vi "Add Round Key.vi"(0 "ExpandedKey(w)":u32[][](array[numeric]), 2 "Nb":i32=4, 7 "State.In":u16[][](array[numeric]), 9 "rnd (0)":i32, 11 "error in":errorcluster) -> (8 "State.Out":u16[][](array[numeric]), 15 "error out":errorcluster)   [LabVIEW 2020, in "Advanced Encryption Standard (AES).lvlib"]
doc: "In the AddRoundKey step, the subkey is combined with the state. For each round, a subkey is derived from the main key using Rijndael's key schedule; each subkey is the same size as the state. The subkey is added by combining each byte of the state with the corresponding byte of the subkey using bitwise XOR.\n\n<inline>"
uses:
  Advanced Encryption Standard (AES).lvlib
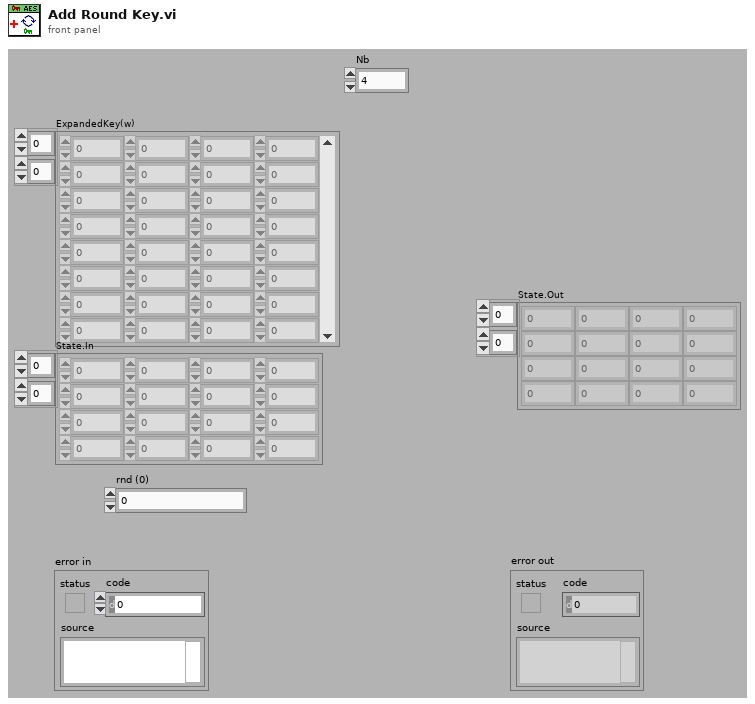
[diagram p1: front panel]
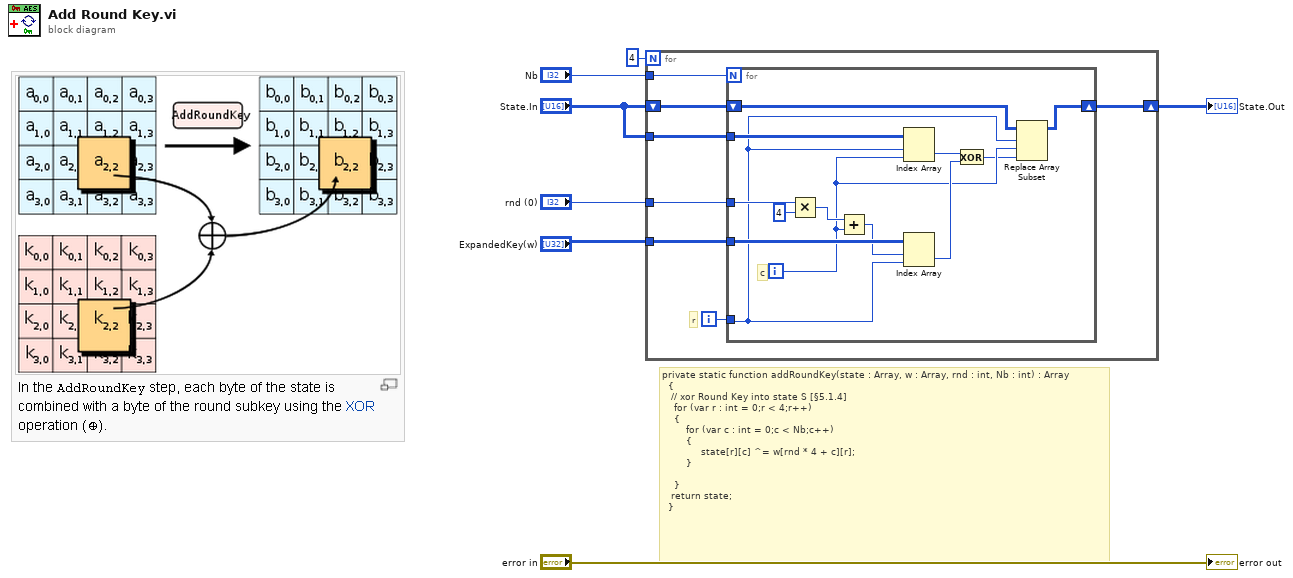
[diagram p0: block diagram]
diagram:
  # "private static function addRoundKey(state : Array, w : Array, rnd : int, Nb : int) : Array \n\t\t{  \n\t\t\t// xor Round Key into state S [§5.1.4]\n\t\t\t\tfor (var r : int = 0;r < 4;r++) \n    {\n\t\t\t\t    for (var c : int = 0;c < Nb;c++) \n\t\t\t\t    {\n\t\t\t\t         state[r][c] ^= w[rnd * 4 + c][r];\n\t\t\t\t    }\n\t\t\t\t\n\t\t\t }\n\t\t\treturn state;\n\t\t}"
  n1 = for {
    N: 4 -> [_]
    tunnel: "State.In" -> [w13]
    tunnel: "ExpandedKey(w)" -> [w12]
    tunnel: "Nb" -> [w11]
    tunnel: "rnd (0)" -> [w10]
    shift-right: [w8] -> w2
    shift-left: "State.In" -> [w9]
    i -> [w14]
    # "r"
    n2 = for {
      N: w11 -> [_]
      tunnel: w14 -> [w19]
      tunnel: w13 -> [w22]
      tunnel: w12 -> [w27]
      tunnel: w10 -> [w26]
      shift-right: [w15] -> w8
      shift-left: w9 -> [w16]
      i -> [w18]
      # "c"
      n3 = Multiply(x=w26, y=4) -> (x*y=w24:i32)
      n4 = Add(x=w24, y=w18) -> (x+y=w23:i32)
      n5 = Index Array(array=w22, index (row)=w19, index (col)=w18) -> (element=w21:u16)
      n6 = Index Array(array=w27, index (row)=w23, index (col)=w19) -> (element=w20:u32)
      n7 = Exclusive Or(1:w20, 2:w21) -> (0:w17:u32)
      n8 = Replace Array Subset(array=w16, new element=w17, index (row)=w19, index (col)=w18) -> (w15:u16[][])
    }
  }
  "State.Out" <- w2
  "error out" <- "error in"
